vi "Init.vi"(8 "error in (no error)":errorcluster, 11 "Coverage Report in":refnum<class "Coverage Report.lvclass">) -> (0 "error out":errorcluster, 3 "Coverage Report out":refnum<class "Coverage Report.lvclass">)   [LabVIEW 2020, in "Coverage Report.lvclass"]
uses:
  Coverage Report.lvclass
  Coverage Report.lvclass/Coverage Report.ctl
  User Interface/Support/Paths.lvlib
  User Interface/Configuration Manager/Configuration Manager.lvclass
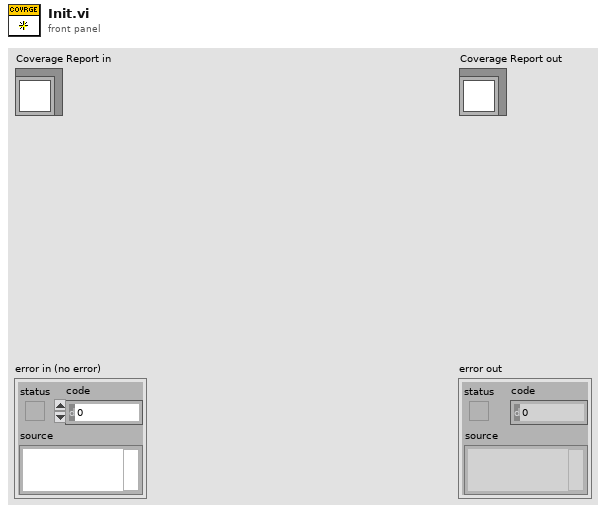
[diagram p1: front panel]
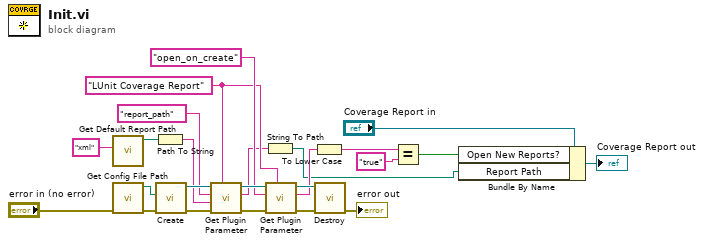
[diagram p0: block diagram]
diagram:
  w9 = "LUnit Coverage Report"
  n1 = call "Get Default Report Path.vi"("File Extension"="xml") -> ("Default Report Path"=w7:path)  [unwired: 9 in, 1 out]
  n2 = call "Get Config File Path.vi"("error in (no error)"="error in (no error)") -> ("error out"=w22:errorcluster, "Config Directory"=w21:path)  [unwired: 9 in]
  n3 = Path To String(path=w7) -> (string=w17:string)
  n4 = call "Create.vi"("error in (no error)"=w22, "configuration file path"=w21) -> ("error out"=w19:errorcluster, "Configuration Manager out"=w23:refnum<class "Configuration Manager.lvclass">)  [unwired: 8 in]
  n5 = call "Get Plugin Parameter.vi"("Plugin"=w9, "error in (no error)"=w19, "Default Value"=w17, "Name"="report_path", "Configuration Manager in"=w23) -> ("error out"=w20:errorcluster, "Value"=w6:string, "Configuration Manager out"=w15:refnum<class "Configuration Manager.lvclass">)  [unwired: 4 in]
  n6 = String To Path(string=w6) -> (path=w1:path)
  n7 = call "Get Plugin Parameter.vi"("Plugin"=w9, "error in (no error)"=w20, "Name"="open_on_create", "Configuration Manager in"=w15) -> ("error out"=w16:errorcluster, "Value"=w12:string, "Configuration Manager out"=w14:refnum<class "Configuration Manager.lvclass">)  [unwired: 5 in]
  n8 = To Lower Case(string=w12) -> (all lower case string=w11:string)
  n9 = call "Destroy.vi"("error in (no error)"=w16, "Configuration Manager In"=w14) -> ("error out"=→"error out":errorcluster)  [unwired: 9 in]
  n10 = Equal?(x=w11, y="true") -> (x = y?=w2:bool)
  n11 = Bundle By Name(cluster="Coverage Report in", "Open New Reports?"=w2, "Report Path"=w1) -> (→"Coverage Report out":refnum<class "Coverage Report.lvclass">)
